vi "ClimberGoToSwitch.vi"(11 "TargetSwitch":T1=enum."2") -> (3 "Done":bool)   [LabVIEW 2012]
uses:
  ClimberLimitSwitches.ctl
  <vilib>/Rock Robotics/WPI/Relay/WPI_RelayValue.ctl
panel:
  in  "Motor Overide":dbl
  in  "Overite Motor":bool
  out "Potentiometer":dbl
  in  "Speed":dbl
  in  "Deadband":dbl
  in  "Off":dbl
  in  "Top":dbl
  in  "4":dbl
  in  "3":dbl
  in  "2":dbl
  in  "1":dbl
  in  "Bottom":dbl
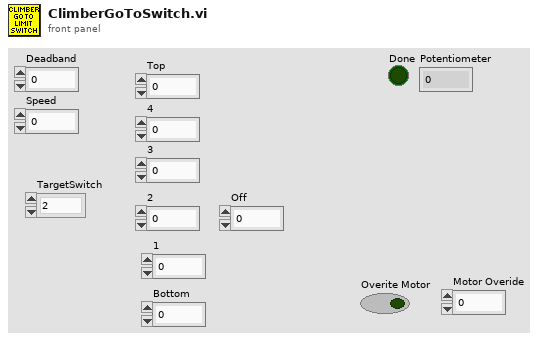
[diagram p1: front panel]
types:
  T1 = typedef "ClimberLimitSwitches.ctl" = enum16{"Off", "Bottom", "1", "2", "3", "4", "Top"}
  T2 = typedef "WPI_AnalogChannelDevRef.ctl" = cluster{"DevStatus":errorcluster, "Analog Module":T3, "Analog Channel":T4}
  T3 = typedef "FPGA_TypedefAnalogModule.ctl" = enum16{"Analog Module 1", "Analog Module 2"}
  T4 = typedef "FPGA_AIChannel.ctl" = enum8{"AI 1", "AI 2", "AI 3", "AI 4", "AI 5", "AI 6", "AI 7", "AI 8", "Invalid"}
  T5 = typedef "WPI_DigitalInputDevRef.ctl" = cluster{"DevStatus":errorcluster, "DIO Channel":T6, "Digital Module":T7}
  T6 = typedef "FPGA_DIOChannel.ctl" = enum8{"DIO 1", "DIO 2", "DIO 3", "DIO 4", "DIO 5", "DIO 6", "DIO 7", "DIO 8", "DIO 9", "DIO 10", "DIO 11", "DIO 12", "DIO 13", "DIO 14", "Invalid"}
  T7 = typedef "FPGA_TypedefDigitalModule.ctl" = enum16{"Digital Module 1", "Digital Module 2"}
  T8 = typedef "WPI_RelayValue.ctl" = enum16{"Off", "On", "Forward", "Reverse"}
  T9 = typedef "WPI_MotorControlDeviceRef.ctl" = cluster{"DeviceStatus":errorcluster, "Type":enum16{"PWM", "CAN"}, "PWM":cluster{"Digital Module":T7, "PWM Channel":T10, "DeadBand":T11}, "CAN":cluster{"Device Number":u8, "Control Mode":T12, "Semaphore":T13, "Max Vout":dbl}, "Invert":bool, "TransformRef":T14, "InvTransformRef":T14}
  T10 = typedef "FPGA_DIOPWMChannel.ctl" = enum8{"PWM 1", "PWM 2", "PWM 3", "PWM 4", "PWM 5", "PWM 6", "PWM 7", "PWM 8", "PWM 9", "PWM 10", "Invalid"}
  T11 = typedef "WPI_PWMDeadband.ctl" = cluster{"Name":string, "maxPositivePwm":i32, "minPositivePwm":i32, "centerPwm":i32, "maxNegativePwm":i32, "minNegativePwm":i32, "angularRange":u16}
  T12 = typedef "WPI_CANJaguar_ControlMode.ctl" = enum8{"Percent VBus", "Current", "Speed", "Position", "Voltage"}
  T13 = typedef "Semaphore RefNum" = refnum<k1>
  T14 = typedef "WPI_PWMTransform_ConPane.ctl" = refnum<vi>
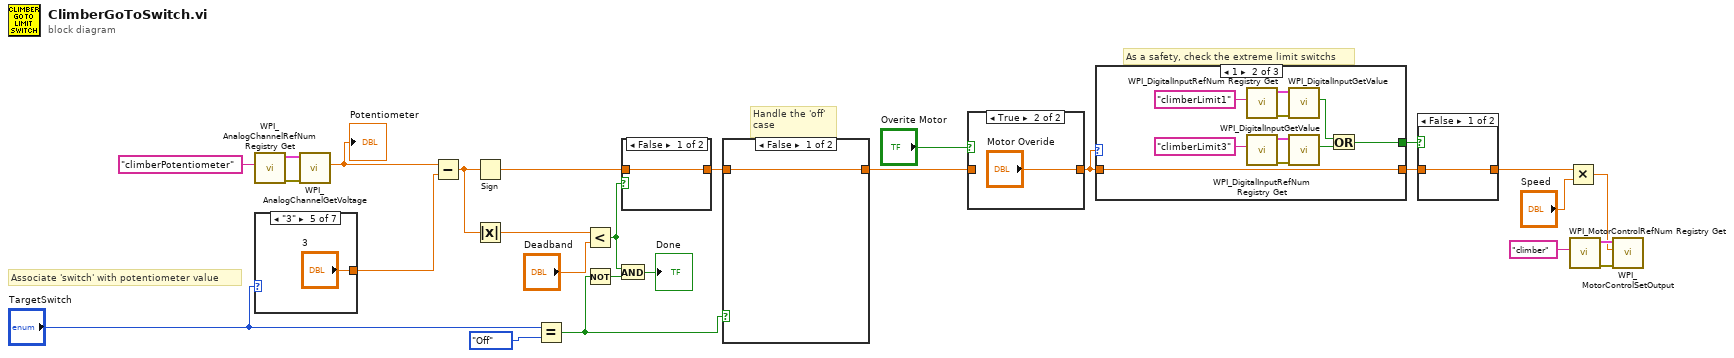
[diagram p0: block diagram]
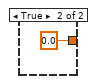
[diagram p3: hidden frame]
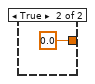
[diagram p4: hidden frame]
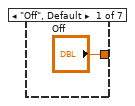
[diagram p5: hidden frame]
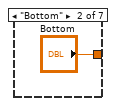
[diagram p6: hidden frame]
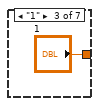
[diagram p7: hidden frame]
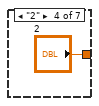
[diagram p8: hidden frame]
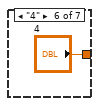
[diagram p9: hidden frame]
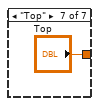
[diagram p10: hidden frame]
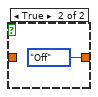
[diagram p11: hidden frame]
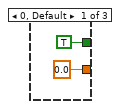
[diagram p12: hidden frame]
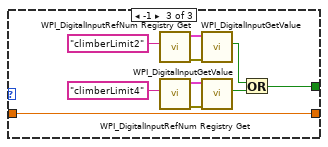
[diagram p13: hidden frame]
diagram:
  # "Handle the 'off'\ncase"
  # "Associate 'switch' with potentiometer value"
  # "As a safety, check the extreme limit switchs"
  n1 = call <vilib>:"WPI_AnalogChannelRefNum Registry Get.vi"("refnum name"="climberPotentiometer") -> ("error out"=w24:errorcluster, "AIDeviceRef"=w23:T2)  [unwired: 9 in]
  n2 = case shown="\"3\"" "TargetSwitch" {
    tunnel: ["Off" "Bottom" "1" "2" "3" "4" "Top"] -> w21
    frame "Off", Default {
    }
    frame "Bottom" {
    }
    frame "1" {
    }
    frame "2" {
    }
    frame "3" {
    }
    frame "4" {
    }
    frame "Top" {
    }
  }
  n3 = call <vilib>:"WPI_AnalogChannelGetVoltage.vi"("error in (no error)"=w24, "AIDeviceRef"=w23) -> ("Voltage"=w22:dbl)  [unwired: 7 in, 2 out]
  "Potentiometer" <- w22
  n4 = Subtract(x=w22, y=w21) -> (x-y=w18:dbl)
  n5 = Sign(1:w18) -> (0:w17:dbl)
  n6 = Absolute Value(x=w18) -> (abs(x)=w20:dbl)
  n7 = Equal?(x="TargetSwitch", y=ClimberLimitSwitches."Off" ("TargetSwitch")) -> (x = y?=w5:bool)
  n8 = Less?(x=w20, y="Deadband") -> (x < y?=w14:bool)
  n9 = Not(x=w5) -> (.not. x?=w13:bool)
  n10 = And(x=w14, y=w13) -> (x .and. y?=→"Done":bool)
  n11 = case shown="False" w14 {
    tunnel: [w35 0.0] -> w4
    tunnel: w17 -> [w35 _]
    frame False {
    }
    frame True {
    }
  }
  n12 = case shown="False" w5 {
    tunnel: [w37 0.0] -> w3
    tunnel: w4 -> [w37 _]
    frame False {
    }
    frame True {
    }
  }
  n13 = case shown="True" "Overite Motor" {
    tunnel: w3 -> [w39 _]
    tunnel: [w39 "Motor Overide"] -> w2
    frame False {
    }
    frame True {
    }
  }
  n14 = case shown="1" w2 {
    tunnel: [TRUE ("Value") w45 w55] -> w27
    tunnel: [0.0 w49 w60] -> w25
    tunnel: w2 -> [_ w49 w60]
    frame 0, Default {
    }
    frame 1 {
      n15 = call <vilib>:"WPI_DigitalInputRefNum Registry Get.vi"("refnum name"="climberLimit1") -> ("error out"=w52:errorcluster, "DigitalInputDevRef"=w51:T5)  [unwired: 9 in]
      n16 = call <vilib>:"WPI_DigitalInputRefNum Registry Get.vi"("refnum name"="climberLimit3") -> ("error out"=w48:errorcluster, "DigitalInputDevRef"=w47:T5)  [unwired: 9 in]
      n17 = call <vilib>:"WPI_DigitalInputGetValue.vi"("error in (no error)"=w52, "DigitalInputDevRef"=w51) -> ("Value"=w44:bool)  [unwired: 7 in, 2 out]
      n18 = call <vilib>:"WPI_DigitalInputGetValue.vi"("error in (no error)"=w48, "DigitalInputDevRef"=w47) -> ("Value"=w43:bool)  [unwired: 7 in, 2 out]
      n19 = Or(x=w44, y=w43) -> (x .or. y?=w45:bool)
    }
    frame -1 {
      n20 = call <vilib>:"WPI_DigitalInputRefNum Registry Get.vi"("refnum name"="climberLimit2") -> ("error out"=w59:errorcluster, "DigitalInputDevRef"=w62:T5)  [unwired: 9 in]
      n21 = call <vilib>:"WPI_DigitalInputRefNum Registry Get.vi"("refnum name"="climberLimit4") -> ("error out"=w56:errorcluster, "DigitalInputDevRef"=w58:T5)  [unwired: 9 in]
      n22 = call <vilib>:"WPI_DigitalInputGetValue.vi"("error in (no error)"=w59, "DigitalInputDevRef"=w62) -> ("Value"=w54:bool)  [unwired: 7 in, 2 out]
      n23 = call <vilib>:"WPI_DigitalInputGetValue.vi"("error in (no error)"=w56, "DigitalInputDevRef"=w58) -> ("Value"=w53:bool)  [unwired: 7 in, 2 out]
      n24 = Or(x=w54, y=w53) -> (x .or. y?=w55:bool)
    }
  }
  n25 = case shown="False" w27 {
    tunnel: [w63 WPI_RelayValue."Off" ("RelayValue")] -> w10
    tunnel: w25 -> [w63 _]
    frame False {
    }
    frame True {
    }
  }
  n26 = Multiply(x=w10, y="Speed") -> (x*y=w6:dbl)
  n27 = call <vilib>:"WPI_MotorControlRefNum Registry Get.vi"("refnum name"="climber") -> ("error out"=w8:errorcluster, "MotorControlDevRef"=w7:T9)  [unwired: 9 in]
  n28 = call <vilib>:"WPI_MotorControlSetOutput.vi"("error in (no error)"=w8, "Output"=w6, "MotorControlDevRef"=w7) -> ()  [unwired: 6 in, 3 out]
